vi "Read from Hardware.vi"(8 "error in":errorcluster, 10 "Values in":dbl[](array[numeric]), 11 "Tx UDP Execution Unit in":refnum<class "Tx UDP Execution Unit.lvclass">) -> (0 "error out":errorcluster, 2 "Values out":dbl[](array[numeric]), 3 "Tx UDP Execution Unit out":refnum<class "Tx UDP Execution Unit.lvclass">)   [LabVIEW 2020, in "AIM ARINC 664 Engine.lvlib" / "Implementation.lvlib" / "Tx UDP Execution Unit.lvclass"]
uses:
  Tx UDP Execution Unit.lvclass
  Tx UDP Execution Unit.lvclass/Tx UDP Execution Unit.ctl
  <instrlib>/AIM GmbH/_AIM 664/AIM664LV.lvlib
  <vilib>/Utility/SystemLogging/NI_SystemLogging.lvlib
panel:
  out "IndexCycleCounts":u32[](array[numeric])
  out "CurrentIndexes":u32[](array[numeric])
  out "MsgCounts":u32[](array[numeric])
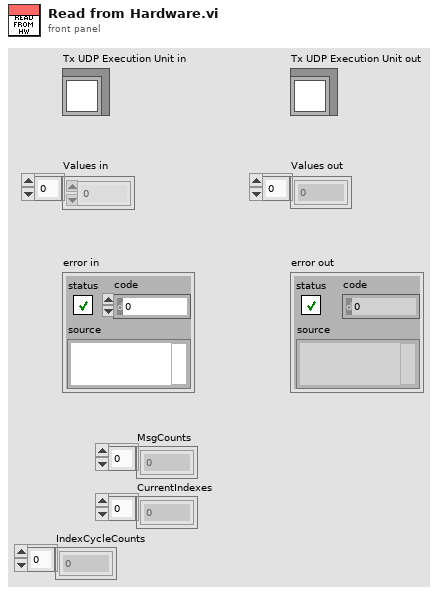
[diagram p1: front panel]
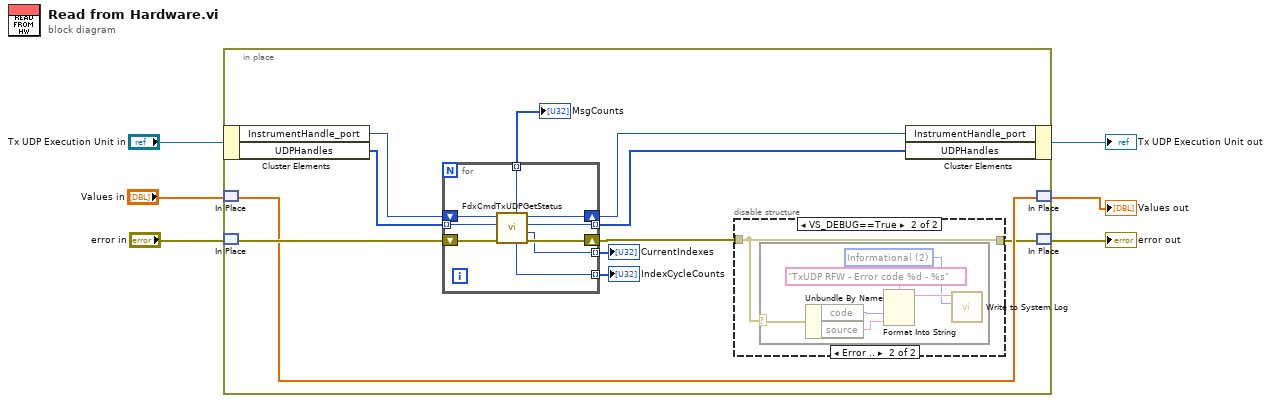
[diagram p0: block diagram]
diagram:
  n1 = in-place {
    n2 = in-place-cluster #1("Tx UDP Execution Unit in") -> ("InstrumentHandle_port"=w17:u32, "UDPHandles"=w16:u32[])
    n3 = in-place-match #2("Values in") -> (w9:dbl[])
    n4 = in-place-match #3("error in") -> (w15:errorcluster)
    n5 = for {
      tunnel: w16 -> [w33] mode=indexing
      shift-right: [w30] -> w14
      shift-left: w17 -> [w34]
      shift-right: [w31] -> w8
      shift-left: w15 -> [w32]
      tunnel: [w29] -> w13 mode=indexing
      tunnel: [w28] -> w12 mode=indexing
      tunnel: [w27] -> w11 mode=indexing
      tunnel: [w26] -> w10 mode=indexing
      n6 = call <instrlib>:"FdxCmdTxUDPGetStatus.vi"("error in"=w32, "UdpHandle"=w33, "InstrumentHandle"=w34) -> ("error out"=w31:errorcluster, "CurrentIndex"=w27:u32, "UdpHandleOut"=w29:u32, "InstrumentHandle"=w30:u32, "IndexCycleCount"=w26:u32, "MsgCount"=w28:u32)  [unwired: 3 in]
    }
    "MsgCounts" <- w12
    "CurrentIndexes" <- w11
    "IndexCycleCounts" <- w10
    n7 = disable-structure shown="VS_DEBUG==True" {
      disable-tunnel: w8 -> [w18 w19]
      disable-tunnel: [w18 w19] -> w7
      frame condition #0 (active) {
      }
      frame condition #1 {
        n8 = case shown="Error .." w19 {
          selector: w19 -> [_ w20]
          frame No Error {
          }
          frame Error {
            w23 = 2 items=["Error", "Warning", "Informational"] ("severity")
            n9 = Unbundle By Name(w20) -> ("code"=w22:i32, "source"=w21:string)
            n10 = Format Into String(format string="TxUDP RFW - Error code %d - %s", w22, w21) -> (resulting string=w24:string)  [unwired: 2 in, 1 out]
            n11 = call <vilib>:"Write to System Log.vi"("severity"=w23, "message"=w24) -> ()  [unwired: 9 in, 1 out]
          }
        }
      }
    }
    n12 = in-place-cluster #1("InstrumentHandle_port"=w14, "UDPHandles"=w13) -> (→"Tx UDP Execution Unit out":refnum<class "Tx UDP Execution Unit.lvclass">)
    n13 = in-place-match #2(w9) -> (→"Values out":dbl[])
    n14 = in-place-match #3(w7) -> (→"error out":errorcluster)
  }
